vi "Init_Images.vi"() -> (3 "Image_Dsts_Out":T1[](array[typedef]))   [LabVIEW 2011]
uses:
  <vilib>/vision/Image Controls.llb/IMAQ Image.ctl
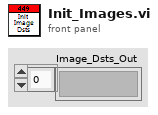
[diagram p1: front panel]
types:
  T1 = typedef "IMAQ Image.ctl" = refnum<image>
  T2 = typedef "Image Type" = u32
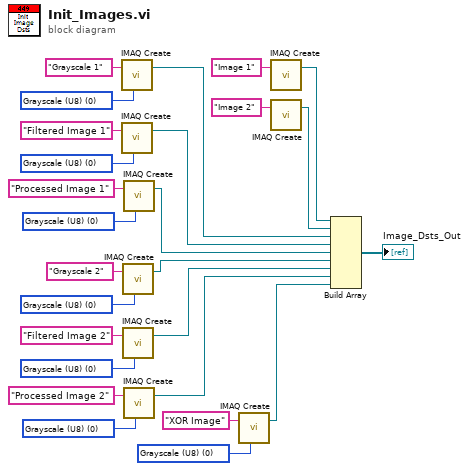
[diagram p0: block diagram]
diagram:
  w14 = T2 0 items=["Grayscale (U8)", "Grayscale (I16)", "Grayscale (SGL)", "Complex (CSG)", "RGB (U32)", "HSL (U32)", "RGB (U64)", "Grayscale (U16)"] ("Image Type")
  w16 = T2 0 items=["Grayscale (U8)", "Grayscale (I16)", "Grayscale (SGL)", "Complex (CSG)", "RGB (U32)", "HSL (U32)", "RGB (U64)", "Grayscale (U16)"] ("Image Type")
  w17 = T2 0 items=["Grayscale (U8)", "Grayscale (I16)", "Grayscale (SGL)", "Complex (CSG)", "RGB (U32)", "HSL (U32)", "RGB (U64)", "Grayscale (U16)"] ("Image Type")
  w20 = T2 0 items=["Grayscale (U8)", "Grayscale (I16)", "Grayscale (SGL)", "Complex (CSG)", "RGB (U32)", "HSL (U32)", "RGB (U64)", "Grayscale (U16)"] ("Image Type")
  w21 = T2 0 items=["Grayscale (U8)", "Grayscale (I16)", "Grayscale (SGL)", "Complex (CSG)", "RGB (U32)", "HSL (U32)", "RGB (U64)", "Grayscale (U16)"] ("Image Type")
  w24 = T2 0 items=["Grayscale (U8)", "Grayscale (I16)", "Grayscale (SGL)", "Complex (CSG)", "RGB (U32)", "HSL (U32)", "RGB (U64)", "Grayscale (U16)"] ("Image Type")
  w25 = T2 0 items=["Grayscale (U8)", "Grayscale (I16)", "Grayscale (SGL)", "Complex (CSG)", "RGB (U32)", "HSL (U32)", "RGB (U64)", "Grayscale (U16)"] ("Image Type")
  n1 = call "IMAQ Create"("Image Name"="Grayscale 1", "Image Type"=w17) -> ("New Image"=w8:T1)  [unwired: 3 in, 1 out]
  n2 = call "IMAQ Create"("Image Name"="Filtered Image 1", "Image Type"=w21) -> ("New Image"=w7:T1)  [unwired: 3 in, 1 out]
  n3 = call "IMAQ Create"("Image Name"="Grayscale 2", "Image Type"=w16) -> ("New Image"=w5:T1)  [unwired: 3 in, 1 out]
  n4 = call "IMAQ Create"("Image Name"="Filtered Image 2", "Image Type"=w20) -> ("New Image"=w4:T1)  [unwired: 3 in, 1 out]
  n5 = call "IMAQ Create"("Image Name"="Processed Image 1", "Image Type"=w25) -> ("New Image"=w6:T1)  [unwired: 3 in, 1 out]
  n6 = call "IMAQ Create"("Image Name"="Processed Image 2", "Image Type"=w24) -> ("New Image"=w3:T1)  [unwired: 3 in, 1 out]
  n7 = call "IMAQ Create"("Image Name"="XOR Image", "Image Type"=w14) -> ("New Image"=w2:T1)  [unwired: 3 in, 1 out]
  n8 = call "IMAQ Create"("Image Name"="Image 1") -> ("New Image"=w10:T1)  [unwired: 4 in, 1 out]
  n9 = call "IMAQ Create"("Image Name"="Image 2") -> ("New Image"=w9:T1)  [unwired: 4 in, 1 out]
  n10 = Build Array(w10, w9, w8, w7, w6, w5, w4, w3, w2) -> (→"Image_Dsts_Out":T1[])
